vi "StressControl.vi"(0 "Function":T3, 1 "Speed (°/s)":dbl=4.0 min=0.0 max=4.0 format="%.6f", 3 "VISA In":refnum<visa-resource-name>="COM4", 5 "Destination (°)":dbl min=-2000000000.0 max=2000000000.0 format="%.6f", 9 "Axis":i32=1 min=1 max=3, 11 "error in (no error)":errorcluster, 12 "Motion":u16(ring) items=["Absolute", "Relative"], 13 "StressControl Notifications":T2, 14 "Motor Refnums":T4) -> (6 "Position (°)":dbl=25.0 format="%.6g", 15 "error out":errorcluster)   [LabVIEW 2014]
uses:
  StressControl Refnums.ctl
  StressControl Functions.ctl
  StressControl Notifiers.ctl
  support/Instrument Status.ctl
  support/Instrument Status State.ctl
  <instrlib>/Newport ESP301/Newport ESP301.lvlib
panel:
  out "Instrument Status":T1
  in  "stop":bool
  # "LICENSED MATERIALS – PROPERTY OF IBM\nCopyright IBM Corp. 2016,\nALL RIGHTS RESERVED"
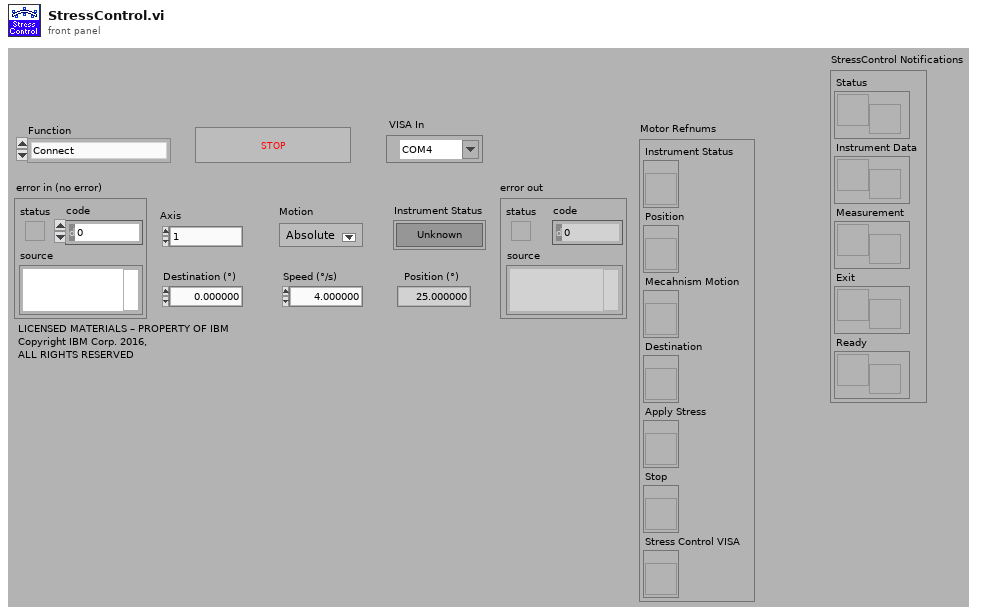
[diagram p1: front panel]
types:
  T1 = typedef "Instrument Status.ctl" = bool
  T2 = typedef "StressControl Notifiers.ctl" = cluster{"Status":refnum<notifier>, "Instrument Data":refnum<notifier>, "Measurement":refnum<notifier>, "Exit":refnum<notifier>, "Ready":refnum<notifier>}
  T3 = typedef "StressControl Functions.ctl" = enum16{"Connect", "Configure", "Get position", "Move", "Disconnect", "Update Refnums"}
  T4 = typedef "StressControl Refnums.ctl" = cluster{"Instrument Status":refnum<vi>, "Position":refnum<vi>, "Mecahnism Motion":refnum<vi>, "Destination":refnum<vi>, "Apply Stress":refnum<vi>, "Stop":refnum<vi>, "Stress Control VISA":refnum<vi>}
  T5 = typedef "Instrument Status State.ctl" = enum16{"Unknown", "Idle", "Standby", "Configuring", "Measuring", "Moving", "Disconnected"}
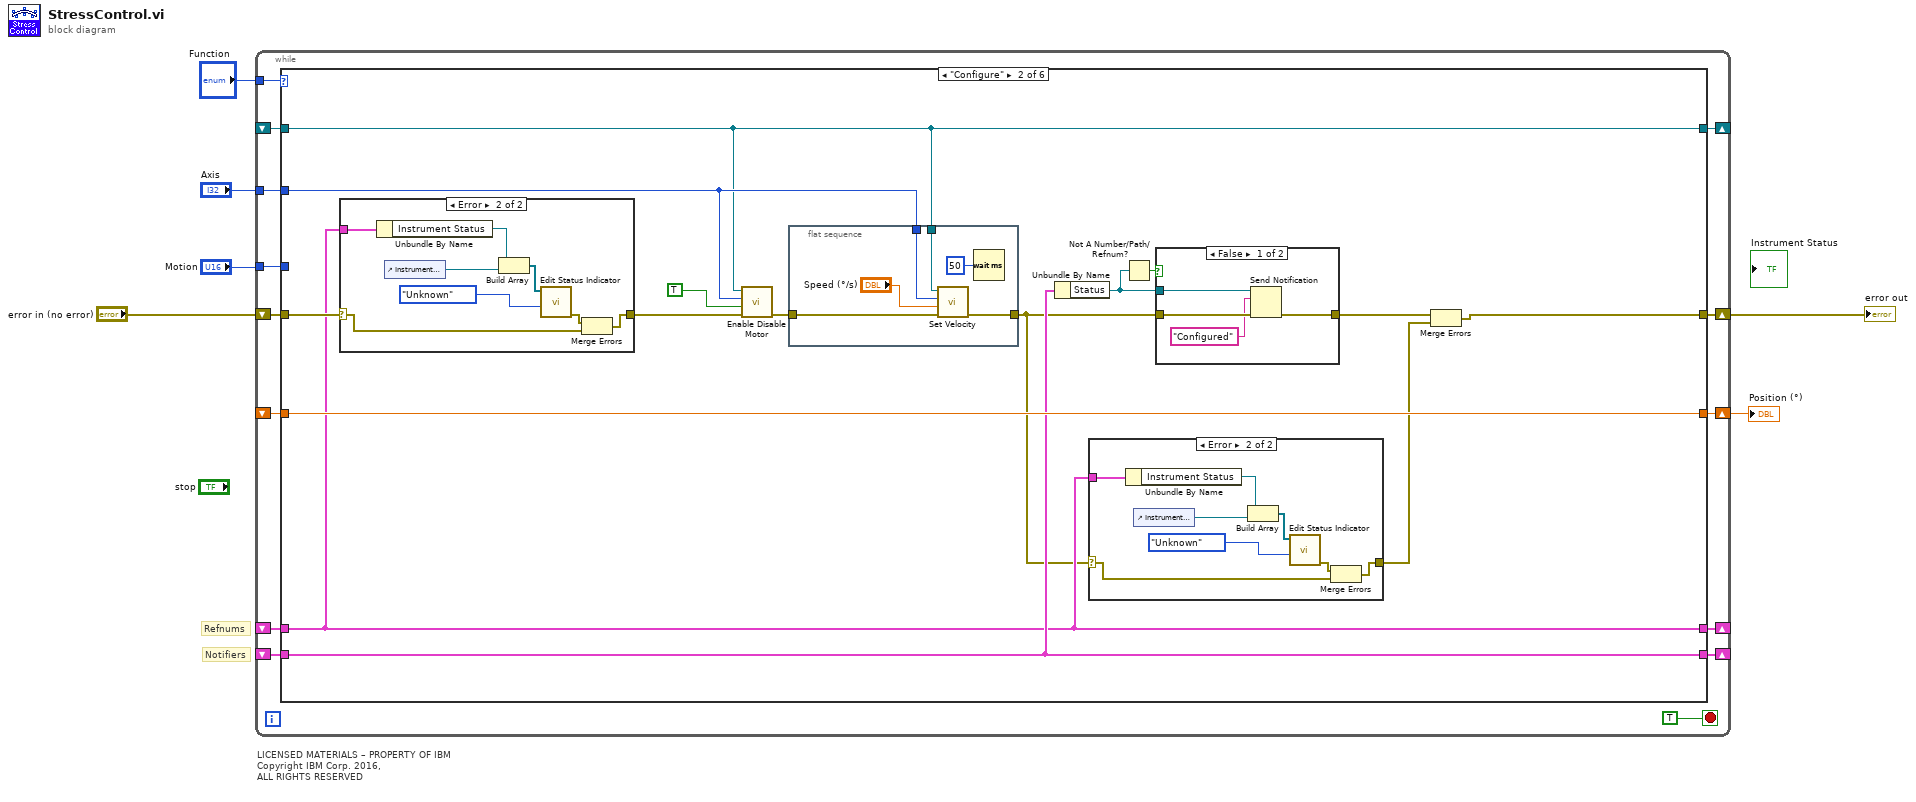
[diagram p0: block diagram]
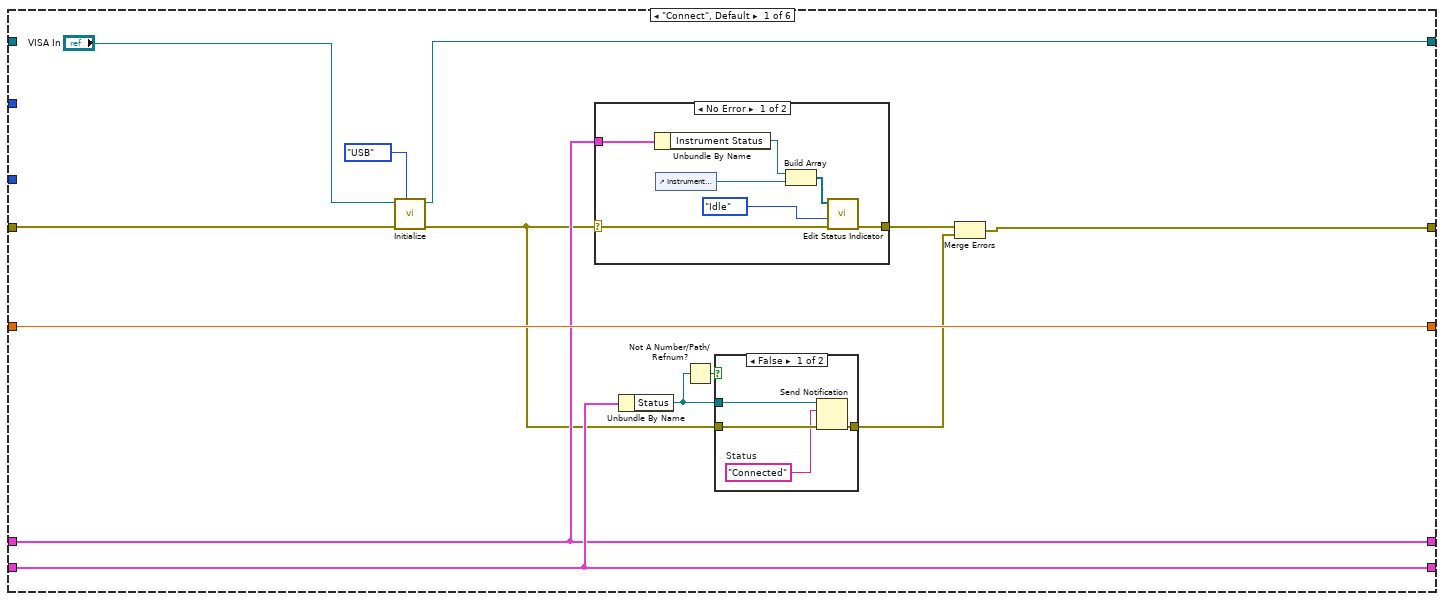
[diagram p2: hidden frame]
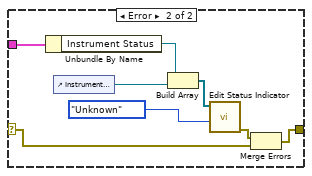
[diagram p3: hidden frame]
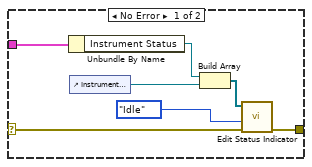
[diagram p5: hidden frame]
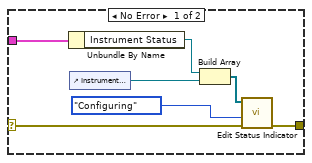
[diagram p6: hidden frame]
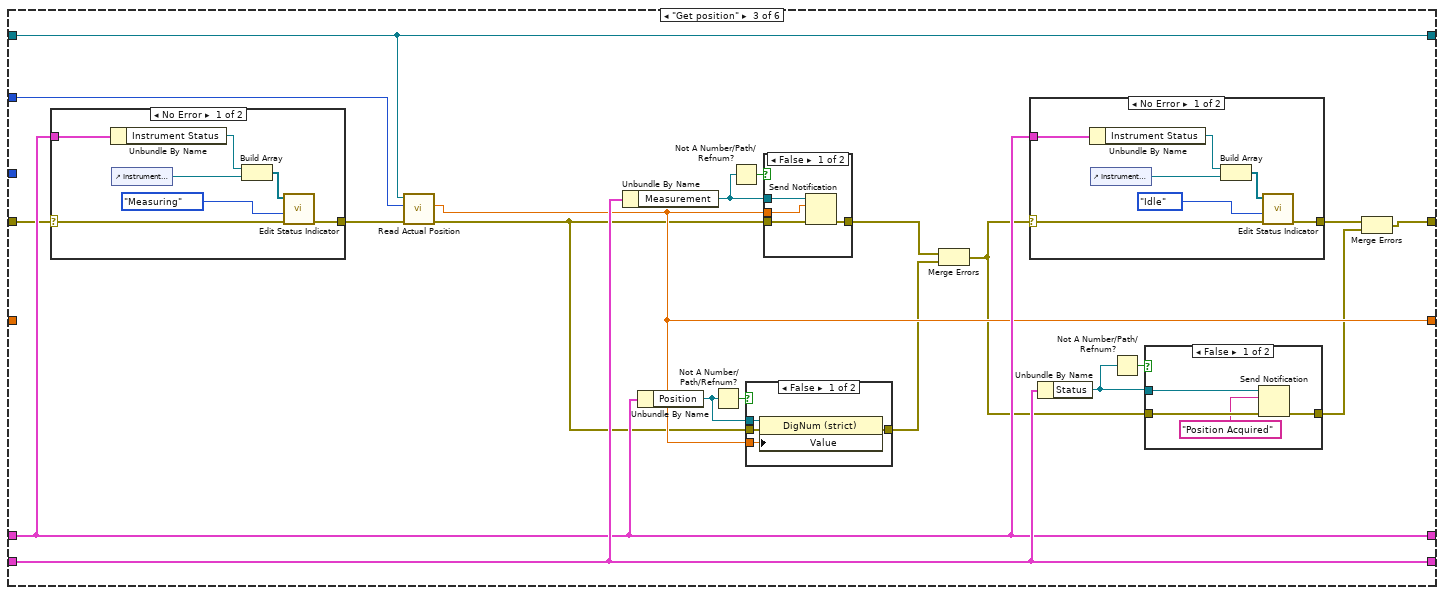
[diagram p8: hidden frame]
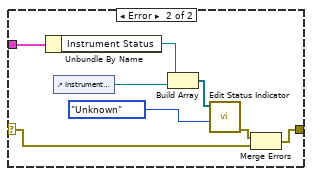
[diagram p10: hidden frame]
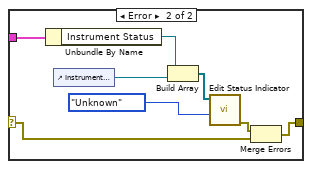
[diagram p11: hidden frame]
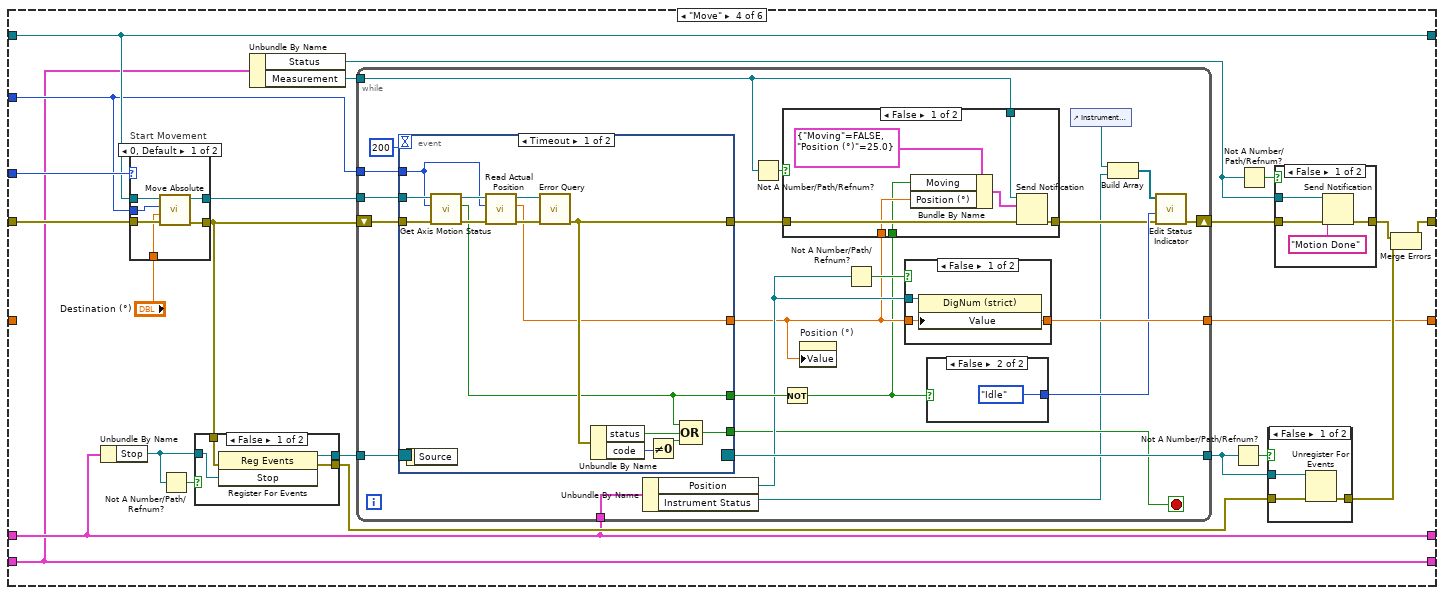
[diagram p14: hidden frame]
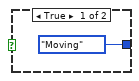
[diagram p16: hidden frame]
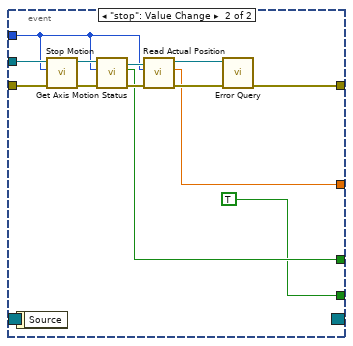
[diagram p18: hidden frame]
diagram:
  # "LICENSED MATERIALS – PROPERTY OF IBM\nCopyright IBM Corp. 2016,\nALL RIGHTS RESERVED"
  # "Notifiers"
  # "Refnums"
  n1 = while {
    shift-right: [w19] -> _
    shift-left: _ -> [w18]
    tunnel: "Function" -> [w17]
    tunnel: "Motion" -> [w15]
    tunnel: "Axis" -> [w16]
    shift-right: [w13] -> w6
    shift-left: "error in (no error)" -> [w14]
    shift-right: [w12] -> _
    shift-left: _ -> [w11]
    shift-right: [w10] -> w1
    shift-left: _ -> [w9]
    shift-right: [w8] -> _
    shift-left: _ -> [w7]
    stop <- TRUE stop-if-true
    n2 = case shown="\"Configure\"" w17 {
      tunnel: [w31 w63 w129 w190 w296 w325] -> w19
      tunnel: w18 -> [_ w63 w129 w190 w296 w325]
      tunnel: w16 -> [_ w64 w128 w185 _ _]
      tunnel: w15 -> [_ _ _ w197 _ _]
      tunnel: w14 -> [w33 w59 w118 w189 w297 w320]
      tunnel: [w22 w56 w110 w192 w289 w318] -> w13
      tunnel: [w25 w58 w122 w184 w290 "Motor Refnums"] -> w12
      tunnel: w11 -> [w25 w58 w122 w184 w290 _]
      tunnel: [w30 w68 w121 w182 w295 w323] -> w10
      tunnel: w9 -> [w30 w68 _ _ w295 w323]
      tunnel: [w29 w67 w124 w181 w294 "StressControl Notifications"] -> w8
      tunnel: w7 -> [w29 w67 w124 w181 w294 _]
      frame "Connect", Default {
        n3 = call <instrlib>:"Initialize.vi"("VISA resource name"="VISA In", "error in (no error)"=w33, "Serial Link (RS232)"=enum16{"RS232", "USB"}."USB") -> ("VISA resource name out"=w31:refnum<visa-resource-name>, "error out"=w23:errorcluster)  [unwired: 2 in, 4 out]
        n4 = case shown="No Error" w23 {
          selector: w23 -> [w39 w45]
          tunnel: [w38 w44] -> w24
          tunnel: w25 -> [w34 w42]
          frame No Error {
            n5 = Unbundle By Name(w34) -> ("Instrument Status"=w35:refnum<vi>)
            n6 = control-ref of="Instrument Status"() -> (w37:refnum<vi>)
            n7 = Build Array(w35, w37) -> (w36:refnum<vi>[])
            n8 = call "Edit Status Indicator.vi"("error in (no error)"=w39, "State"=Instrument_Status_State."Idle", "Instrument Status Refnum"=w36) -> ("error out"=w38:errorcluster)  [unwired: 1 in, 7 out]
          }
          frame Error {
            n9 = Unbundle By Name(w42) -> ("Instrument Status"=w41:refnum<vi>)
            n10 = control-ref of="Instrument Status"() -> (w47:refnum<vi>)
            n11 = Build Array(w41, w47) -> (w46:refnum<vi>[])
            n12 = call "Edit Status Indicator.vi"("State"=Instrument_Status_State."Unknown", "Instrument Status Refnum"=w46) -> ("error out"=w43:errorcluster)  [unwired: 2 in, 7 out]
            n13 = Merge Errors(w43, w45) -> (w44:errorcluster)
          }
        }
        n14 = Unbundle By Name(w29) -> ("Status"=w28:refnum<notifier>)
        n15 = Not A Number/Path/Refnum?(number/path/refnum=w28) -> (NaN/Path/Refnum?=w27:bool)
        n16 = case shown="False" w27 {
          tunnel: w28 -> [w52 _]
          tunnel: w23 -> [w51 w53]
          tunnel: [w50 w53] -> w21
          frame False {
            w49 = "Connected"  # Status
            n17 = Send Notification(notification=w49, notifier=w52, error in (no error)=w51) -> (error out=w50:errorcluster)  [unwired: 1 out]
          }
          frame True {
          }
        }
        n18 = Merge Errors(w24, w21) -> (w22:errorcluster)
      }
      frame "Configure" {
        n19 = case shown="Error" w59 {
          selector: w59 -> [w95 w101]
          tunnel: [w94 w100] -> w57
          tunnel: w58 -> [w90 w98]
          frame No Error {
            n20 = Unbundle By Name(w90) -> ("Instrument Status"=w91:refnum<vi>)
            n21 = control-ref of="Instrument Status"() -> (w93:refnum<vi>)
            n22 = Build Array(w91, w93) -> (w92:refnum<vi>[])
            n23 = call "Edit Status Indicator.vi"("error in (no error)"=w95, "State"=Instrument_Status_State."Configuring", "Instrument Status Refnum"=w92) -> ("error out"=w94:errorcluster)  [unwired: 1 in, 7 out]
          }
          frame Error {
            n24 = Unbundle By Name(w98) -> ("Instrument Status"=w97:refnum<vi>)
            n25 = control-ref of="Instrument Status"() -> (w103:refnum<vi>)
            n26 = Build Array(w97, w103) -> (w102:refnum<vi>[])
            n27 = call "Edit Status Indicator.vi"("State"=Instrument_Status_State."Unknown", "Instrument Status Refnum"=w102) -> ("error out"=w99:errorcluster)  [unwired: 2 in, 7 out]
            n28 = Merge Errors(w99, w101) -> (w100:errorcluster)
          }
        }
        n29 = call <instrlib>:"Enable Disable Motor.vi"("error in (no error)"=w57, "Action (F - OFF)"=TRUE, "Axis (1)"=w64, "VISA resource name"=w63) -> ("error out"=w61:errorcluster)  [unwired: 3 out]
        n30 = flat-sequence {
          tunnel: [w74] -> w54
          tunnel: w64 -> [w72]
          tunnel: w63 -> [w71]
          tunnel: w61 -> [w70]
          frame #0 {
            n31 = call <instrlib>:"Set Velocity.vi"("error in (no error)"=w70, "Velocity (units/s)"="Speed (°/s)", "Axis (1)"=w72, "VISA resource name"=w71) -> ("error out"=w74:errorcluster)  [unwired: 3 out]
            n32 = Wait (ms)(milliseconds to wait=u32 50) -> ()  [unwired: 1 out]
          }
        }
        n33 = Unbundle By Name(w67) -> ("Status"=w66:refnum<notifier>)
        n34 = case shown="Error" w54 {
          selector: w54 -> [w80 w86]
          tunnel: [w79 w85] -> w60
          tunnel: w58 -> [w75 w82]
          frame No Error {
            n35 = Unbundle By Name(w75) -> ("Instrument Status"=w76:refnum<vi>)
            n36 = control-ref of="Instrument Status"() -> (w78:refnum<vi>)
            n37 = Build Array(w76, w78) -> (w77:refnum<vi>[])
            n38 = call "Edit Status Indicator.vi"("error in (no error)"=w80, "State"=Instrument_Status_State."Idle", "Instrument Status Refnum"=w77) -> ("error out"=w79:errorcluster)  [unwired: 1 in, 7 out]
          }
          frame Error {
            n39 = Unbundle By Name(w82) -> ("Instrument Status"=w83:refnum<vi>)
            n40 = control-ref of="Instrument Status"() -> (w88:refnum<vi>)
            n41 = Build Array(w83, w88) -> (w87:refnum<vi>[])
            n42 = call "Edit Status Indicator.vi"("State"=Instrument_Status_State."Unknown", "Instrument Status Refnum"=w87) -> ("error out"=w84:errorcluster)  [unwired: 2 in, 7 out]
            n43 = Merge Errors(w84, w86) -> (w85:errorcluster)
          }
        }
        n44 = Not A Number/Path/Refnum?(number/path/refnum=w66) -> (NaN/Path/Refnum?=w65:bool)
        n45 = case shown="False" w65 {
          tunnel: w54 -> [w108 w109]
          tunnel: [w107 w109] -> w55
          tunnel: w66 -> [w106 _]
          frame False {
            n46 = Send Notification(notification="Configured", notifier=w106, error in (no error)=w108) -> (error out=w107:errorcluster)  [unwired: 1 out]
          }
          frame True {
          }
        }
        n47 = Merge Errors(w55, w60) -> (w56:errorcluster)
      }
      frame "Get position" {
        n48 = case shown="No Error" w118 {
          selector: w118 -> [w155 w161]
          tunnel: [w154 w160] -> w117
          tunnel: w122 -> [w150 w157]
          frame No Error {
            n49 = Unbundle By Name(w150) -> ("Instrument Status"=w151:refnum<vi>)
            n50 = control-ref of="Instrument Status"() -> (w153:refnum<vi>)
            n51 = Build Array(w151, w153) -> (w152:refnum<vi>[])
            n52 = call "Edit Status Indicator.vi"("error in (no error)"=w155, "State"=Instrument_Status_State."Measuring", "Instrument Status Refnum"=w152) -> ("error out"=w154:errorcluster)  [unwired: 1 in, 7 out]
          }
          frame Error {
            n53 = Unbundle By Name(w157) -> ("Instrument Status"=w158:refnum<vi>)
            n54 = control-ref of="Instrument Status"() -> (w163:refnum<vi>)
            n55 = Build Array(w158, w163) -> (w162:refnum<vi>[])
            n56 = call "Edit Status Indicator.vi"("State"=Instrument_Status_State."Unknown", "Instrument Status Refnum"=w162) -> ("error out"=w159:errorcluster)  [unwired: 2 in, 7 out]
            n57 = Merge Errors(w159, w161) -> (w160:errorcluster)
          }
        }
        n58 = call <instrlib>:"Read Actual Position.vi"("error in (no error)"=w117, "Axis (1)"=w128, "VISA resource name"=w129) -> ("error out"=w115:errorcluster, "Position (units)"=w121:dbl)  [unwired: 3 out]
        n59 = Unbundle By Name(w124) -> ("Measurement"=w126:refnum<notifier>)
        n60 = Unbundle By Name(w122) -> ("Position"=w119:refnum<vi>)
        n61 = Not A Number/Path/Refnum?(number/path/refnum=w119) -> (NaN/Path/Refnum?=w120:bool)
        n62 = Not A Number/Path/Refnum?(number/path/refnum=w126) -> (NaN/Path/Refnum?=w127:bool)
        n63 = case shown="False" w120 {
          tunnel: w121 -> [w132 _]
          tunnel: w119 -> [w133 _]
          tunnel: w115 -> [w131 w134]
          tunnel: [w130 w134] -> w116
          frame False {
            n64 = property class="DigNum (strict)"(reference=w133, error in=w131, "Value"=w132) -> (error out=w130:errorcluster)  [unwired: 1 out]
          }
          frame True {
          }
        }
        n65 = case shown="False" w127 {
          tunnel: [w173 w174] -> w112
          tunnel: w126 -> [w172 _]
          tunnel: w115 -> [w171 w174]
          tunnel: w121 -> [w170 _]
          frame False {
            n66 = Send Notification(notification=w170, notifier=w172, error in (no error)=w171) -> (error out=w173:errorcluster)  [unwired: 1 out]
          }
          frame True {
          }
        }
        n67 = Merge Errors(w112, w116) -> (w114:errorcluster)
        n68 = case shown="No Error" w114 {
          selector: w114 -> [w140 w146]
          tunnel: [w139 w145] -> w111
          tunnel: w122 -> [w136 w143]
          frame No Error {
            n69 = Unbundle By Name(w136) -> ("Instrument Status"=w135:refnum<vi>)
            n70 = control-ref of="Instrument Status"() -> (w138:refnum<vi>)
            n71 = Build Array(w135, w138) -> (w137:refnum<vi>[])
            n72 = call "Edit Status Indicator.vi"("error in (no error)"=w140, "State"=Instrument_Status_State."Idle", "Instrument Status Refnum"=w137) -> ("error out"=w139:errorcluster)  [unwired: 1 in, 7 out]
          }
          frame Error {
            n73 = Unbundle By Name(w143) -> ("Instrument Status"=w142:refnum<vi>)
            n74 = control-ref of="Instrument Status"() -> (w148:refnum<vi>)
            n75 = Build Array(w142, w148) -> (w147:refnum<vi>[])
            n76 = call "Edit Status Indicator.vi"("State"=Instrument_Status_State."Unknown", "Instrument Status Refnum"=w147) -> ("error out"=w144:errorcluster)  [unwired: 2 in, 7 out]
            n77 = Merge Errors(w144, w146) -> (w145:errorcluster)
          }
        }
        n78 = Unbundle By Name(w124) -> ("Status"=w123:refnum<notifier>)
        n79 = Not A Number/Path/Refnum?(number/path/refnum=w123) -> (NaN/Path/Refnum?=w125:bool)
        n80 = case shown="False" w125 {
          tunnel: [w168 w169] -> w113
          tunnel: w123 -> [w167 _]
          tunnel: w114 -> [w166 w169]
          frame False {
            n81 = Send Notification(notification="Position Acquired", notifier=w167, error in (no error)=w166) -> (error out=w168:errorcluster)  [unwired: 1 out]
          }
          frame True {
          }
        }
        n82 = Merge Errors(w111, w113) -> (w110:errorcluster)
      }
      frame "Move" {
        n83 = Unbundle By Name(w184) -> ("Stop"=w194:refnum<vi>)
        n84 = case "Start Movement" shown="0, Default" w197 {
          tunnel: w190 -> [w280 w284]
          tunnel: [w279 w286] -> w188
          tunnel: w189 -> [w278 w283]
          tunnel: [w277 w285] -> w187
          tunnel: w185 -> [w276 w282]
          tunnel: "Destination (°)" -> [w275 w281]
          frame 0, Default {
            n85 = call <instrlib>:"Move Absolute.vi"("error in (no error)"=w278, "Position (0 units)"=w275, "Axis (1)"=w276, "VISA resource name"=w280) -> ("error out"=w277:errorcluster, "VISA resource name out"=w279:refnum<visa-resource-name>)  [unwired: 2 out]
          }
          frame 1 {
            n86 = call <instrlib>:"Move Relative.vi"("error in (no error)"=w283, "Position (0 units)"=w281, "Axis (1)"=w282, "VISA resource name"=w284) -> ("error out"=w285:errorcluster, "VISA resource name out"=w286:refnum<visa-resource-name>)  [unwired: 2 out]
          }
        }
        n87 = Not A Number/Path/Refnum?(number/path/refnum=w194) -> (NaN/Path/Refnum?=w196:bool)
        n88 = case shown="False" w196 {
          tunnel: w194 -> [w273 _]
          tunnel: [w272 _] -> w186
          tunnel: w187 -> [w271 w274]
          tunnel: [w270 w274] -> w193
          frame False {
            n89 = register-events(error in=w271, w273) -> (reference out=w272:refnum<event-registration>, error out=w270:errorcluster)  [unwired: 1 in]
          }
          frame True {
          }
        }
        n90 = Unbundle By Name(w181) -> ("Status"=w177:refnum<notifier>, "Measurement"=w180:refnum<notifier>)
        n91 = while "Polling until the destination is reached or Error occurs" {
          tunnel: w185 -> [w214]
          tunnel: w188 -> [w225]
          tunnel: w186 -> [w219]
          tunnel: [w218] -> w183
          tunnel: w184 -> [w220]
          tunnel: [w213] -> w182
          tunnel: w180 -> [w211]
          shift-right: [w205] -> w179
          shift-left: w187 -> [w224]
          stop <- w215 stop-if-true
          n92 = event shown="[0] Timeout" {
            selector: w219 -> [_ _]
            dyn-events: [_ _] -> w218
            timeout: 200 -> [_ _]
            tunnel: [w245 w260] -> w222
            tunnel: [w240 w259] -> w212
            tunnel: [w241 TRUE] -> w215
            tunnel: [w237 w254] -> w221
            tunnel: w225 -> [w239 w252]
            tunnel: w224 -> [w238 w251]
            tunnel: w214 -> [w236 w250]
            event Timeout {
              n93 = event-data() -> ()  [unwired: 2 out]
              n94 = call <instrlib>:"Get Axis Motion Status.vi"("error in (no error)"=w238, "Axis (1)"=w236, "VISA resource name"=w239) -> ("error out"=w249:errorcluster, "Motion Done"=w237:bool, "VISA resource name out"=w248:refnum<visa-resource-name>)  [unwired: 2 out]
              n95 = call <instrlib>:"Read Actual Position.vi"("error in (no error)"=w249, "Axis (1)"=w236, "VISA resource name"=w248) -> ("error out"=w247:errorcluster, "Position (units)"=w240:dbl, "VISA resource name out"=w246:refnum<visa-resource-name>)  [unwired: 2 out]
              n96 = call <instrlib>:"Error Query.vi"("error in (no error)"=w247, "VISA resource name"=w246) -> ("error out"=w245:errorcluster)  [unwired: 5 out]
              n97 = Unbundle By Name(w245) -> ("status"=w243:bool, "code"=w244:i32)
              n98 = Not Equal To 0?(x=w244) -> (x != 0?=w242:bool)
              n99 = Compound Arithmetic op=OR(w237, w243, w242) -> (w241:bool)
            }
            event "stop": Value Change {
              n100 = event-data() -> ()  [unwired: 2 out]
              n101 = call <instrlib>:"Stop Motion.vi"("error in (no error)"=w251, "Axis (1)"=w250, "VISA resource name"=w252) -> ("error out"=w255:errorcluster, "VISA resource name out"=w258:refnum<visa-resource-name>)  [unwired: 1 in, 2 out]
              n102 = call <instrlib>:"Get Axis Motion Status.vi"("error in (no error)"=w255, "Axis (1)"=w250, "VISA resource name"=w258) -> ("error out"=w256:errorcluster, "Motion Done"=w254:bool, "VISA resource name out"=w257:refnum<visa-resource-name>)  [unwired: 2 out]
              n103 = call <instrlib>:"Read Actual Position.vi"("error in (no error)"=w256, "Axis (1)"=w250, "VISA resource name"=w257) -> ("error out"=w261:errorcluster, "Position (units)"=w259:dbl, "VISA resource name out"=w262:refnum<visa-resource-name>)  [unwired: 2 out]
              n104 = call <instrlib>:"Error Query.vi"("error in (no error)"=w261, "VISA resource name"=w262) -> ("error out"=w260:errorcluster)  [unwired: 5 out]
            }
          }
          n105 = Unbundle By Name(w220) -> ("Position"=w216:refnum<vi>, "Instrument Status"=w204:refnum<vi>)
          n106 = Not A Number/Path/Refnum?(number/path/refnum=w211) -> (NaN/Path/Refnum?=w210:bool)
          n107 = Not(x=w221) -> (.not. x?=w203:bool)
          n108 = case shown="False" w210 {
            tunnel: w222 -> [w234 w235]
            tunnel: [w233 w235] -> w206
            tunnel: w211 -> [w232 _]
            tunnel: w212 -> [w230 _]
            tunnel: w203 -> [w229 _]
            frame False {
              n109 = Bundle By Name(cluster=cluster{"Moving":bool, "Position (°)":dbl} {"Moving"=FALSE, "Position (°)"=25.0}, "Moving"=w229, "Position (°)"=w230) -> (w228:cluster{"Moving":bool, "Position (°)":dbl})
              n110 = Send Notification(notification=w228, notifier=w232, error in (no error)=w234) -> (error out=w233:errorcluster)  [unwired: 1 out]
            }
            frame True {
            }
          }
          n111 = property on="Position (°)" class="DigNum (strict)"("Value"=w212) -> ()  [unwired: 2 in, 2 out]
          n112 = Not A Number/Path/Refnum?(number/path/refnum=w216) -> (NaN/Path/Refnum?=w217:bool)
          n113 = case shown="False" w217 {
            tunnel: w212 -> [w263 w265]
            tunnel: w216 -> [w264 _]
            tunnel: [w263 w265] -> w213
            frame False {
              n114 = property class="DigNum (strict)"(reference=w264, "Value"=w263) -> ()  [unwired: 1 in, 2 out]
            }
            frame True {
            }
          }
          n115 = case shown="False" w203 {
            tunnel: [Instrument_Status_State."Moving" ("State") Instrument_Status_State."Idle" ("State")] -> w209
            frame True {
            }
            frame False {
            }
          }
          n116 = control-ref of="Instrument Status"() -> (w208:refnum<vi>)
          n117 = Build Array(w208, w204) -> (w207:refnum<vi>[])
          n118 = call "Edit Status Indicator.vi"("error in (no error)"=w206, "State"=w209, "Instrument Status Refnum"=w207) -> ("error out"=w205:errorcluster)  [unwired: 1 in, 7 out]
        }
        n119 = Not A Number/Path/Refnum?(number/path/refnum=w183) -> (NaN/Path/Refnum?=w195:bool)
        n120 = Not A Number/Path/Refnum?(number/path/refnum=w177) -> (NaN/Path/Refnum?=w176:bool)
        n121 = case shown="False" w195 {
          tunnel: w193 -> [w268 w269]
          tunnel: [w267 w269] -> w191
          tunnel: w183 -> [w266 _]
          frame False {
            n122 = Unregister For Events(event registration refnum=w266, error in=w268) -> (error out=w267:errorcluster)
          }
          frame True {
          }
        }
        n123 = case shown="False" w176 {
          tunnel: w179 -> [w201 w202]
          tunnel: [w200 w202] -> w178
          tunnel: w177 -> [w199 _]
          frame False {
            n124 = Send Notification(notification="Motion Done", notifier=w199, error in (no error)=w201) -> (error out=w200:errorcluster)  [unwired: 1 out]
          }
          frame True {
          }
        }
        n125 = Merge Errors(w178, w191) -> (w192:errorcluster)
      }
      frame "Disconnect" {
        n126 = call <instrlib>:"Close.vi"("error in (no error)"=w297, "VISA resource name"=w296) -> ("error out"=w288:errorcluster)  [unwired: 9 out]
        n127 = Unbundle By Name(w294) -> ("Status"=w292:refnum<notifier>)
        n128 = case shown="Error" w288 {
          selector: w288 -> [w303 w309]
          tunnel: [w302 w308] -> w291
          tunnel: w290 -> [w298 w306]
          frame No Error {
            n129 = Unbundle By Name(w298) -> ("Instrument Status"=w299:refnum<vi>)
            n130 = control-ref of="Instrument Status"() -> (w301:refnum<vi>)
            n131 = Build Array(w299, w301) -> (w300:refnum<vi>[])
            n132 = call "Edit Status Indicator.vi"("error in (no error)"=w303, "State"=Instrument_Status_State."Disconnected", "Instrument Status Refnum"=w300) -> ("error out"=w302:errorcluster)  [unwired: 1 in, 7 out]
          }
          frame Error {
            n133 = Unbundle By Name(w306) -> ("Instrument Status"=w305:refnum<vi>)
            n134 = control-ref of="Instrument Status"() -> (w311:refnum<vi>)
            n135 = Build Array(w305, w311) -> (w310:refnum<vi>[])
            n136 = call "Edit Status Indicator.vi"("State"=Instrument_Status_State."Unknown", "Instrument Status Refnum"=w310) -> ("error out"=w307:errorcluster)  [unwired: 2 in, 7 out]
            n137 = Merge Errors(w307, w309) -> (w308:errorcluster)
          }
        }
        n138 = Not A Number/Path/Refnum?(number/path/refnum=w292) -> (NaN/Path/Refnum?=w293:bool)
        n139 = case shown="False" w293 {
          tunnel: w288 -> [w316 w317]
          tunnel: [w315 w317] -> w287
          tunnel: w292 -> [w314 _]
          frame False {
            n140 = Send Notification(notification="Disconnected", notifier=w314, error in (no error)=w316) -> (error out=w315:errorcluster)  [unwired: 1 out]
          }
          frame True {
          }
        }
        n141 = Merge Errors(w287, w291) -> (w289:errorcluster)
      }
      frame "Update Refnums" {
        n142 = Unbundle By Name("StressControl Notifications") -> ("Status"=w322:refnum<notifier>)
        n143 = Not A Number/Path/Refnum?(number/path/refnum=w322) -> (NaN/Path/Refnum?=w321:bool)
        n144 = case shown="False" w321 {
          tunnel: w320 -> [w329 w330]
          tunnel: [w328 w330] -> w318
          tunnel: w322 -> [w327 _]
          frame False {
            n145 = Send Notification(notification="Refnums Updated", notifier=w327, error in (no error)=w329) -> (error out=w328:errorcluster)  [unwired: 1 out]
          }
          frame True {
          }
        }
      }
    }
  }
  "error out" <- w6
  "Position (°)" <- w1
